vi "Request Target Data.vi"(6 "Qualifier":string, 8 "error in":errorcluster, 9 "Data to Request":string, 10 "Instrument":string, 11 "Launcher in":refnum<class "Launcher.lvclass">) -> (0 "error out":errorcluster, 2 "Data":variant, 3 "Launcher out":refnum<class "Launcher.lvclass">)   [LabVIEW 2023, in "Launcher.lvlib" / "Launcher.lvclass"]
uses:
  Library/Launcher.lvclass
  builds/Instruments/Instruments.lvlibp/Instruments Messages/Request Data Msg/Request Data Msg.lvclass
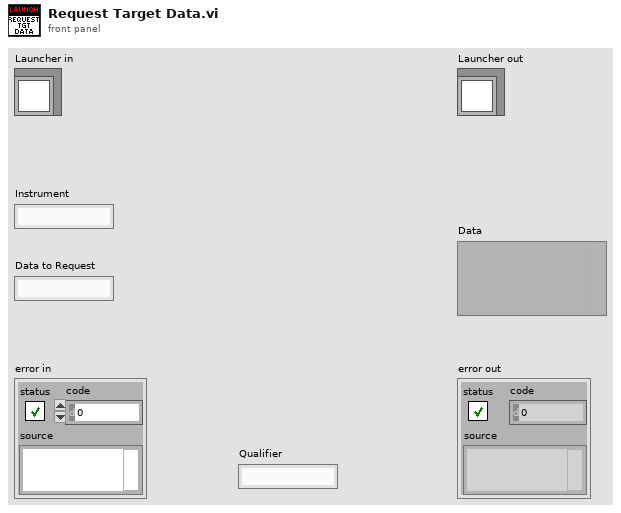
[diagram p1: front panel]
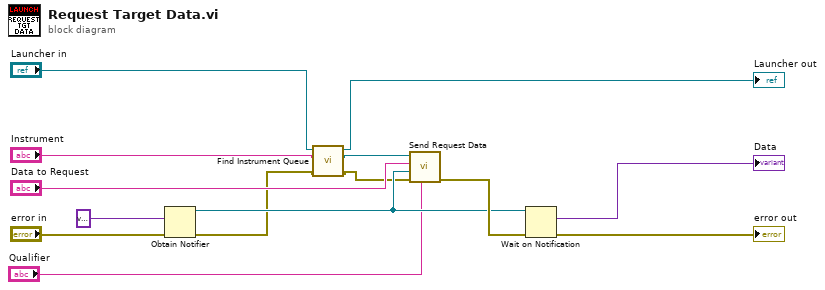
[diagram p0: block diagram]
diagram:
  n1 = Obtain Notifier(notification data type=variant, error in (no error)="error in") -> (notifier out=w11:refnum<notifier>, error out=w4:errorcluster)  [unwired: 2 in, 1 out]
  n2 = call "Find Instrument Queue.vi"("error in"=w4, "Instrument"="Instrument", "Launcher in"="Launcher in") -> ("error out"=w3:errorcluster, "Queue"=w6:refnum<class "Message Enqueuer.lvclass">, "Launcher out"=→"Launcher out":refnum<class "Launcher.lvclass">)  [unwired: 6 in]
  n3 = call "Send Request Data.vi"("Qualifier"="Qualifier", "error in (no error)"=w3, "notifier"=w11, "Data to Send"="Data to Request", "Message Enqueuer"=w6) -> ("error out"=w12:errorcluster)  [unwired: 5 in, 1 out]
  n4 = Wait on Notification(notifier=w11, error in (no error)=w12) -> (notification=→"Data":variant, error out=→"error out":errorcluster)  [unwired: 2 in, 2 out]
